vi "Read ConfigInterface.vi"(11 "Device in":refnum<class "Device.lvclass">) -> (2 "ConfigInterface":refnum<class "ConfigInterface.lvclass">)   [LabVIEW 2019, in "Device.lvclass"]
uses:
  Device.lvclass
  ConfigInterface_class/ConfigInterface.lvclass
  Device.lvclass/Device.ctl
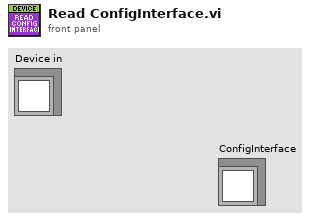
[diagram p1: front panel]
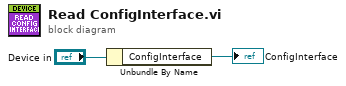
[diagram p0: block diagram]
diagram:
  n1 = Unbundle By Name("Device in") -> ("ConfigInterface"=→"ConfigInterface":refnum<class "ConfigInterface.lvclass">)
